vi "CS4_setpt_rate_chk.vi"(1 "Rate in Range (T/min)":dbl[](array[numeric]), 2 "Set Point":dbl) -> (0 "chk set pt and rate":bool)   [LabVIEW 2012]
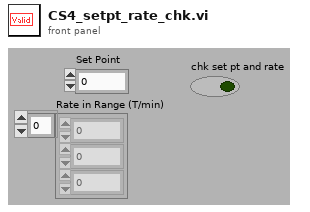
[diagram p1: front panel]
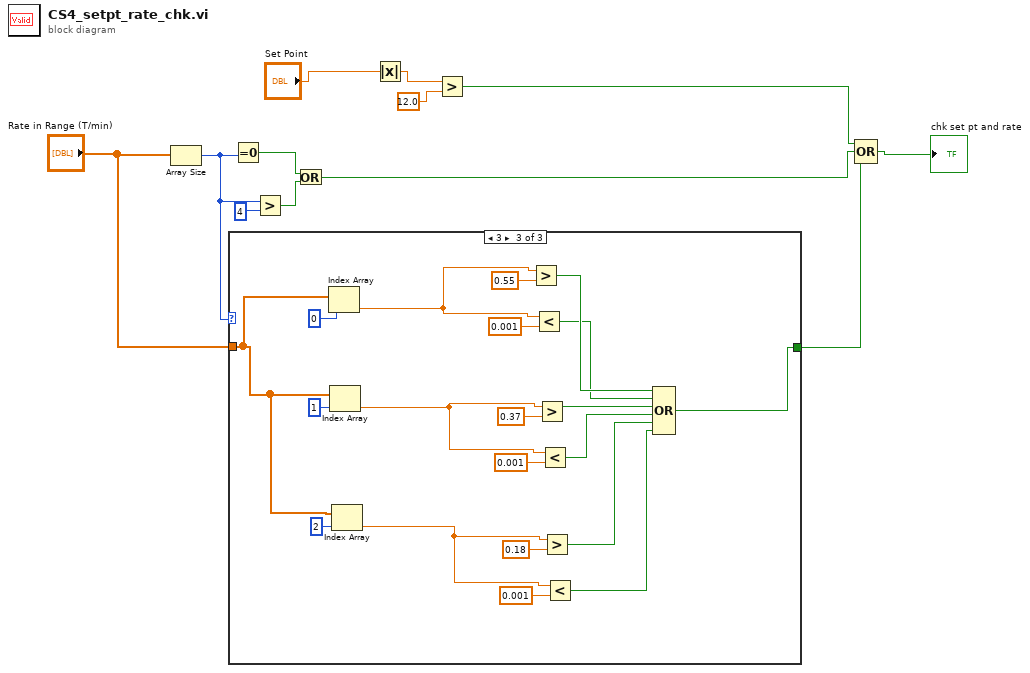
[diagram p0: block diagram]
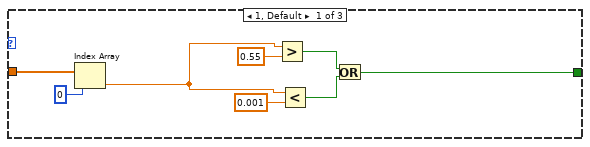
[diagram p2: hidden frame]
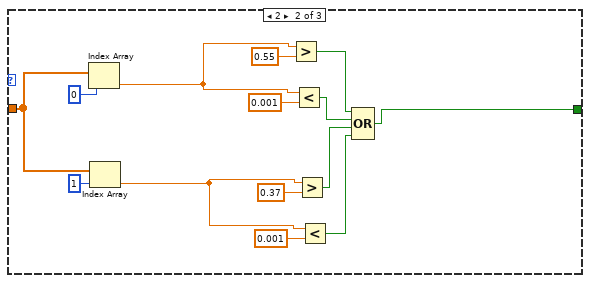
[diagram p3: hidden frame]
diagram:
  n1 = Array Size(array="Rate in Range (T/min)") -> (size(s)=w6:i32)
  n2 = case shown="3" w6 {
    tunnel: "Rate in Range (T/min)" -> [w14 w26 w42]
    tunnel: [w13 w21 w35] -> w1
    frame 1, Default {
      n3 = Index Array(array=w14, index=0) -> (element=w15:dbl)
      n4 = Greater?(x=w15, y=0.55) -> (0:w19:bool)
      n5 = Less?(x=w15, y=0.001) -> (x < y?=w20:bool)
      n6 = Or(x=w19, y=w20) -> (x .or. y?=w13:bool)
    }
    frame 2 {
      n7 = Index Array(array=w26, index=0) -> (element=w31:dbl)
      n8 = Index Array(array=w26, index=1) -> (element=w27:dbl)
      n9 = Greater?(x=w31, y=0.55) -> (0:w25:bool)
      n10 = Less?(x=w31, y=0.001) -> (x < y?=w24:bool)
      n11 = Greater?(x=w27, y=0.37) -> (0:w23:bool)
      n12 = Less?(x=w27, y=0.001) -> (x < y?=w22:bool)
      n13 = Compound Arithmetic op=OR(w25, w24, w23, w22) -> (w21:bool)
    }
    frame 3 {
      n14 = Index Array(array=w42, index=0) -> (element=w51:dbl)
      n15 = Index Array(array=w42, index=1) -> (element=w47:dbl)
      n16 = Index Array(array=w42, index=2) -> (element=w43:dbl)
      n17 = Greater?(x=w51, y=0.55) -> (0:w41:bool)
      n18 = Less?(x=w51, y=0.001) -> (x < y?=w40:bool)
      n19 = Greater?(x=w47, y=0.37) -> (0:w39:bool)
      n20 = Less?(x=w47, y=0.001) -> (x < y?=w38:bool)
      n21 = Greater?(x=w43, y=0.18) -> (0:w37:bool)
      n22 = Less?(x=w43, y=0.001) -> (x < y?=w36:bool)
      n23 = Compound Arithmetic op=OR(w41, w40, w39, w38, w37, w36) -> (w35:bool)
    }
  }
  n24 = Equal To 0?(x=w6) -> (x = 0?=w7:bool)
  n25 = Greater?(x=w6, y=4) -> (0:w8:bool)
  n26 = Or(x=w7, y=w8) -> (x .or. y?=w2:bool)
  n27 = Absolute Value(x="Set Point") -> (abs(x)=w11:dbl)
  n28 = Greater?(x=w11, y=12.0 ("x")) -> (0:w3:bool)
  n29 = Compound Arithmetic op=OR(w3, w2, w1) -> (→"chk set pt and rate":bool)
